vi "Create Plugins.vi"(5 "framework options":T1, 7 "framework configuration":T6, 8 "error in (no error)":errorcluster, 10 "components directory":path, 11 "Framework in":refnum<class "Framework.lvclass">) -> (0 "error out":errorcluster, 1 "Plugin Threads":refnum<class "Plugin Thread.lvclass">[](array[class]), 2 "Plugins":refnum<class "Plugin.lvclass">[](array[class]), 3 "Framework out":refnum<class "Framework.lvclass">)   [LabVIEW 2017, in "DSF Core.lvlib" / "Framework.lvclass"]
uses:
  Framework.lvclass
  Plugin/Plugin.lvclass
  Typedefs/DSF Engine Framework Configuration.ctl
  Typedefs/DSF Engine Plugin Configuration.ctl
  Typedefs/DSF Timing Info.ctl
  Typedefs/DSF Engine Plugin Thread Configuration.ctl
  Typedefs/DSF Settings Info.ctl
  Typedefs/DSF Engine Transfer Group Configuration.ctl
  Typedefs/DSF Direction.ctl
  Typedefs/DSF Engine Transfer Configuration.ctl
  Typedefs/DSF Byte Order.ctl
  Typedefs/DSF Engine Channel Configuration.ctl
  Typedefs/DSF Data Type.ctl
  Typedefs/DSF Timeout Behavior.ctl
  Thread/Plugin/Plugin Thread.lvclass
  Framework Options.ctl
  Typedefs/DSF FIFO Options.ctl
  Thread/DSF Thread Options.ctl
  Typedefs/DSF Plugin Options.ctl
  Typedefs/DSF Performance Options.ctl
  Framework.lvclass/Framework.ctl
  Transceiver/Transceiver.lvclass
  Buffer Converter/Buffer Converter.lvclass
  Framework Status/Framework Status.lvclass/Framework Status.ctl
  Configuration/Required Buffer Size (Plugin).vi
  Configuration/Transfer Group Count (Plugin).vi
  Component Loader/Component Loader.lvclass
  DSF Core.lvlib
  Buffers/Buffers.lvclass
  Transfer Group Status/Status.lvclass
  Framework Status/Framework Status.lvclass
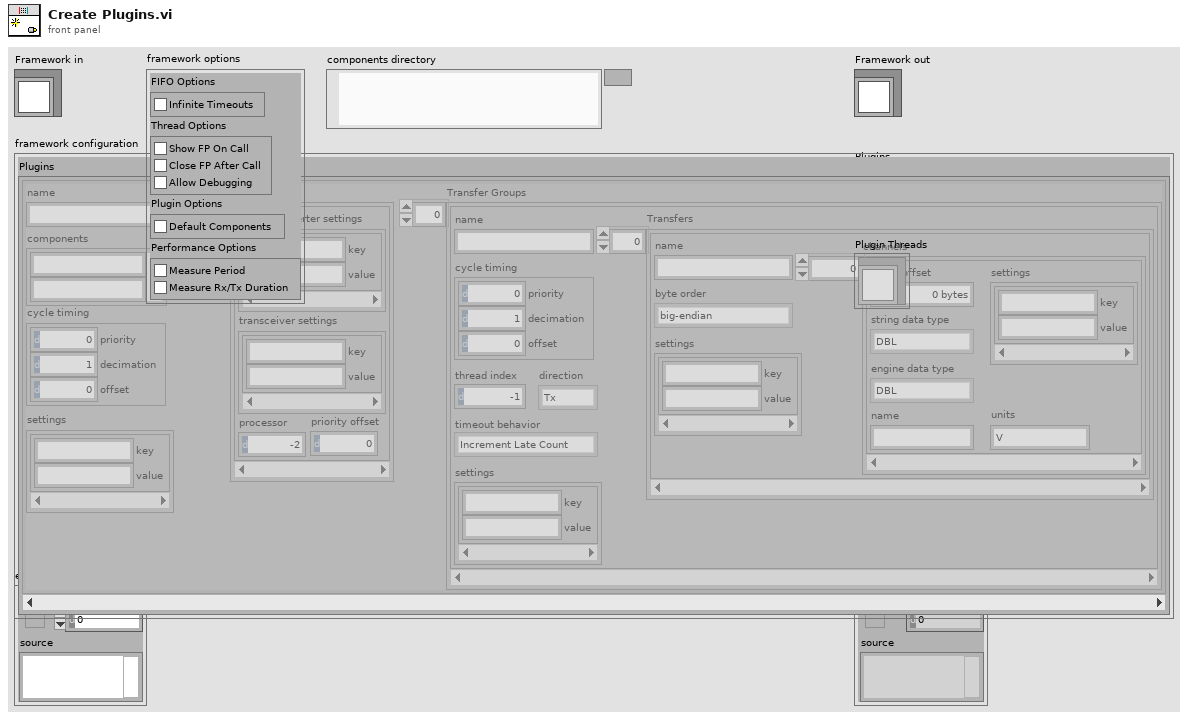
[diagram p1: front panel]
types:
  T1 = typedef "DSF Core.lvlib/Framework.lvclass/Framework Options.ctl" = cluster{"FIFO Options":T2, "Thread Options":T3, "Plugin Options":T4, "Performance Options":T5}
  T2 = typedef "DSF Core.lvlib/DSF FIFO Options.ctl" = cluster{"Infinite Timeouts":bool}
  T3 = typedef "DSF Core.lvlib/DSF Thread Options.ctl" = cluster{"Show FP On Call":bool, "Close FP After Call":bool, "Allow Debugging":bool}
  T4 = typedef "DSF Core.lvlib/DSF Plugin Options.ctl" = cluster{"Default Components":bool}
  T5 = typedef "DSF Core.lvlib/DSF Performance Options.ctl" = cluster{"Measure Period":bool, "Measure Rx/Tx Duration":bool}
  T6 = typedef "DSF Core.lvlib/DSF Engine Framework Configuration.ctl" = cluster{"Plugins":T7[]}
  T7 = typedef "DSF Core.lvlib/DSF Engine Plugin Configuration.ctl" = cluster{"name":string, "components":string[], "cycle timing":T8, "threads":T9[], "Transfer Groups":T11[], "settings":T10}
  T8 = typedef "DSF Core.lvlib/DSF Timing Info.ctl" = cluster{"priority":u64, "decimation":u64, "offset":u64}
  T9 = typedef "DSF Core.lvlib/DSF Engine Plugin Thread Configuration.ctl" = cluster{"buffer converter settings":T10, "transceiver settings":T10, "processor":i32, "priority offset":i16}
  T10 = typedef "DSF Core.lvlib/DSF Settings Info.ctl" = cluster{"key":string, "value":string}[]
  T11 = typedef "DSF Core.lvlib/DSF Engine Transfer Group Configuration.ctl" = cluster{"name":string, "direction":T12, "cycle timing":T8, "thread index":i32, "settings":T10, "Transfers":T13[], "timeout behavior":T17}
  T12 = typedef "DSF Core.lvlib/DSF Direction.ctl" = enum8{"Tx", "Rx"}
  T13 = typedef "DSF Core.lvlib/DSF Engine Transfer Configuration.ctl" = cluster{"name":string, "byte order":T14, "settings":T10, "channels":T15[]}
  T14 = typedef "DSF Core.lvlib/DSF Byte Order.ctl" = enum8{"big-endian", "little-endian"}
  T15 = typedef "DSF Core.lvlib/DSF Engine Channel Configuration.ctl" = cluster{"string offset":u64, "string data type":T16, "engine data type":T16, "name":string, "settings":T10, "units":string}
  T16 = typedef "DSF Core.lvlib/DSF Data Type.ctl" = enum8{"Bool", "SGL", "DBL", "I8", "I16", "I32", "I64", "U8", "U16", "U32", "U64"}
  T17 = typedef "DSF Core.lvlib/DSF Timeout Behavior.ctl" = enum8{"Increment Late Count", "Throw Error"}
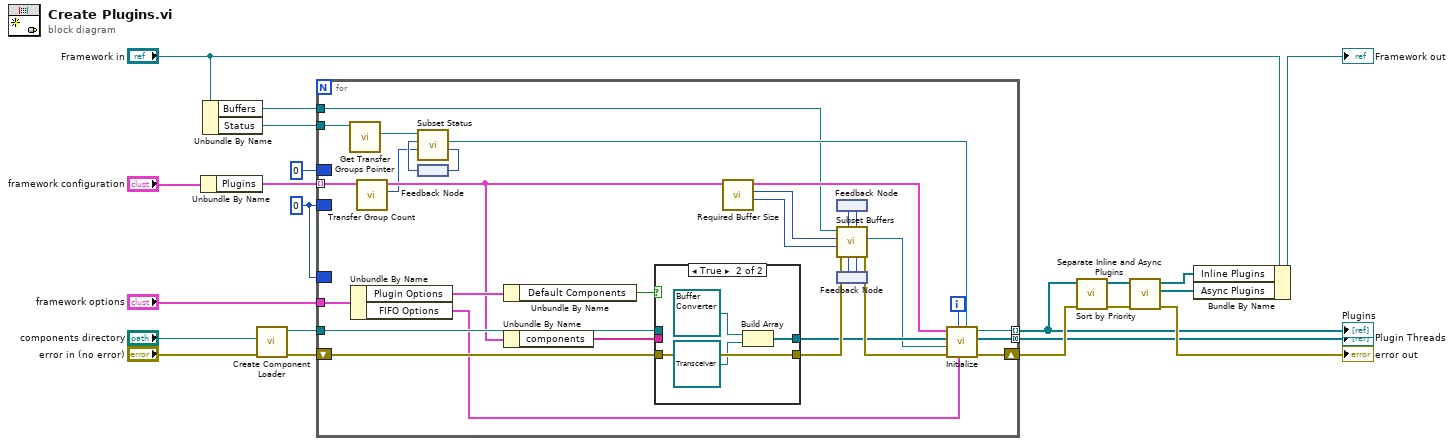
[diagram p0: block diagram]
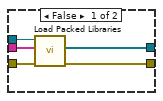
[diagram p2: hidden frame]
diagram:
  w5 = u64 0 ("string buffer offset + size")
  n1 = Unbundle By Name("framework configuration") -> ("Plugins"=w15:T7[])
  n2 = Unbundle By Name("Framework in") -> ("Buffers"=w3:refnum<class "Buffers.lvclass">, "Status"=w4:refnum<class "Framework Status.lvclass">)
  n3 = call "Create Component Loader.vi"("error in (no error)"="error in (no error)", "components directory (default)"="components directory") -> ("error out"=w18:errorcluster, "Component Loader out"=w19:refnum<class "Component Loader.lvclass">)  [unwired: 8 in]
  n4 = for {
    shift-right: [w49] -> w21
    shift-left: w18 -> [w51]
    tunnel: w15 -> [w28] mode=indexing
    tunnel: w19 -> [w52]
    tunnel: [w48] -> w13 mode=indexing
    tunnel: [w34] -> w14 mode=concatenating
    border: w5 -> [_]
    border: w5 -> [_]
    tunnel: "framework options" -> [w39]
    tunnel: w4 -> [w30]
    tunnel: w3 -> [w22]
    border: u64 0 ("group index") -> [_]
    i -> [w47]
    n5 = call "Get Transfer Groups Pointer.vi"("Framework Status in"=w30) -> ("transfer groups pointer"=w29:refnum<class "Status.lvclass">)  [unwired: 9 in, 1 out]
    n6 = Unbundle By Name(w39) -> ("Plugin Options"=w40:T4, "FIFO Options"=w36:T2)
    n7 = call-poly "Transfer Group Count.vi"("Plugin Configuration in"=w28) -> ("transfer group count"=w24:i32, "Plugin Configuration out"=w25:T7)  [unwired: 8 in, 1 out]
    n8 = feedback #1() -> (w26:u64)
    n9 = call "Subset Status.vi"("count (1)"=w24, "index"=w26, "status pointer in"=w29) -> ("index + count"=w27:u64, "subset status pointer"=w23:refnum<class "Status.lvclass">)  [unwired: 5 in, 2 out]
    n10 = feedback-in #1(w27) -> ()
    n11 = Unbundle By Name(w40) -> ("Default Components"=w38:bool)
    n12 = Unbundle By Name(w25) -> ("components"=w50:string[])
    n13 = case shown="True" w38 {
      tunnel: [w57 w61] -> w46
      tunnel: w52 -> [w56 _]
      tunnel: w51 -> [w55 w61]
      tunnel: w50 -> [w54 _]
      tunnel: [w53 w58] -> w35
      frame False {
        n14 = call "Load Packed Libraries.vi"("error in (no error)"=w55, "packed library names"=w54, "Component Loader in"=w56) -> ("error out"=w57:errorcluster, "objects"=w53:refnum<class>[])  [unwired: 6 in, 1 out]
      }
      frame True {
        n15 = Build Array(refnum<class "Buffer Converter.lvclass"> refnum ("DSF Core.lvlib:Buffer Converter"), refnum<class "Transceiver.lvclass"> refnum ("DSF Core.lvlib:Transceiver")) -> (w58:refnum<class>[])
      }
    }
    n16 = call-poly "Required Buffer Size.vi"("Plugin Configuration in"=w25) -> ("total engine buffer size"=w32:u64, "total string buffer size"=w45:u64, "Plugin Configuration out"=w31:T7)  [unwired: 7 in, 1 out]
    n17 = feedback #2() -> (w43:u64)
    n18 = feedback #3() -> (w41:u64)
    n19 = call "Subset Buffers.vi"("inline buffer offset"=w41, "string buffer offset"=w43, "error in (no error)"=w46, "inline buffer size"=w32, "string buffer size"=w45, "Buffers in"=w22) -> ("error out"=w37:errorcluster, "subset Buffers"=w33:refnum<class "Buffers.lvclass">, "inline buffer offset +size"=w42:u64, "string buffer offset + size"=w44:u64)  [unwired: 1 in, 1 out]
    n20 = feedback-in #2(w44) -> ()
    n21 = feedback-in #3(w42) -> ()
    n22 = call "Initialize.vi"("Transfer Group Status"=w23, "FIFO Options"=w36, "id"=w47, "error in (no error)"=w37, "Plugin Buffers"=w33, "component objects"=w35, "Plugin Configuration"=w31) -> ("error out"=w49:errorcluster, "Plugin Threads"=w34:refnum<class "Plugin Thread.lvclass">[], "Plugin out"=w48:refnum<class "Plugin.lvclass">)  [unwired: 2 in]
  }
  "Plugins" <- w13
  "Plugin Threads" <- w14
  n23 = call "Sort by Priority.vi"("error in (no error)"=w21, "Plugins in"=w13) -> ("error out"=w12:errorcluster, "Plugins out"=w7:refnum<class "Plugin.lvclass">[])  [unwired: 8 in]
  n24 = call "Separate Inline and Async Plugins.vi"("error in (no error)"=w12, "Plugins"=w7) -> ("error out"=→"error out":errorcluster, "Async Plugins"=w10:refnum<class "Plugin.lvclass">[], "Inline Plugins"=w11:refnum<class "Plugin.lvclass">[])  [unwired: 7 in]
  n25 = Bundle By Name(cluster="Framework in", "Inline Plugins"=w11, "Async Plugins"=w10) -> (→"Framework out":refnum<class "Framework.lvclass">)
